vi "T7_Read_FLOAT32_Register.vi"(9 "LabJack TestFLOAT32 Register":u16=55124, 10 "Remote Port":u16=502, 11 "Remote IP Address":string="192.168.1.15") -> (6 "Raw Data Read":u16[](array[numeric]), 7 "Read FLOAT32":sgl)   [LabVIEW 2017]
panel:
  # "MB Ethernet Example Master.vi\n\nInstructions\n1.Use Kipling to find your devices IP address & modify the\n\"Remote IP Addres\"\n2. Run this VI\n3. Change value of \"FLOAT32 to Write\" & press \"Write Data\""
  # "TCP Parameters"
  # "Test Write & Read of TEST_UINT32 Register"
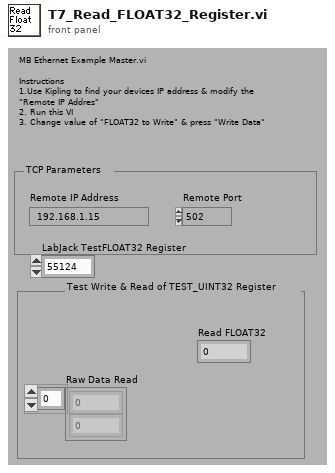
[diagram p1: front panel]
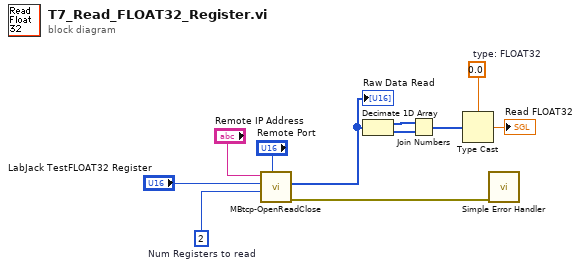
[diagram p0: block diagram]
diagram:
  w8 = sgl 0.0  # type: FLOAT32
  w3 = u16 2  # Num Registers to read
  n1 = call "MBtcp-OpenReadClose.vi"("Port"="Remote Port", "nRegisters"=w3, "RegisterAddr"="LabJack TestFLOAT32 Register", "IP Address"="Remote IP Address") -> ("error out"=w1:errorcluster, "16bitValues"=w2:u16[])  [unwired: 5 in, 1 out]
  "Raw Data Read" <- w2
  n2 = Decimate 1D Array(w2) -> (w11:u16[], w10:u16[])
  n3 = Join Numbers(hi=w11, lo=w10) -> ((hi.lo)=w9:u32[])
  n4 = Type Cast(type=w8, x=w9) -> (*(type *) &x=→"Read FLOAT32":sgl)
  n5 = call <vilib>:"Simple Error Handler.vi"("error in (no error)"=w1) -> ()  [unwired: 1 in, 8 out]
